vi "LabVIEW Time to TAI Time.vi"(5 "LabVIEW Time (s)":timestamp) -> (2 "TAI Time (ns)":u64)   [LabVIEW 2021, in "Time_CIF_U.lvlib"]
doc: "Convert LabVIEW time into TAI time by changing the epoch. TAI time is used as the basis of UTC and is GPS time. It is UTC without leap seconds."
uses:
  Time_CIF_U.lvlib
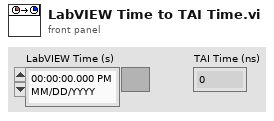
[diagram p1: front panel]
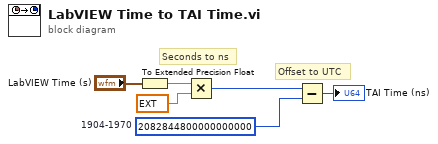
[diagram p0: block diagram]
diagram:
  w5 = u64 2082844800000000000  # 1904-1970
  # "Seconds to ns"
  # "Offset to UTC"
  n1 = To Extended Precision Float(1:"LabVIEW Time (s)") -> (0:w3:ext)
  n2 = Multiply(x=w3, y=ext 1000000000.0) -> (x*y=w4:u64)
  n3 = Subtract(x=w4, y=w5) -> (x-y=→"TAI Time (ns)":u64)
